vi "Verify Checksum.vi"(10 "Message ID":u8 format="%02x", 11 "Data + Checksum":string) -> (3 "Pass":bool)   [LabVIEW 2019]
doc: "Calculates what the checksum of the message should be and verifies it is correct."
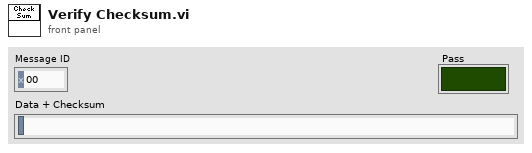
[diagram p1: front panel]
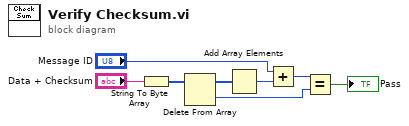
[diagram p0: block diagram]
diagram:
  n1 = String To Byte Array(string="Data + Checksum") -> (unsigned byte array=w4:u8[])
  n2 = Delete From Array(array=w4) -> (deleted portion=w7:u8, array with subset deleted=w5:u8[])  [unwired: 2 in]
  n3 = Add Array Elements(numeric array=w5) -> (sum=w6:u8)
  n4 = Add(x="Message ID", y=w6) -> (x+y=w2:u8)
  n5 = Equal?(x=w2, y=w7) -> (x = y?=→"Pass":bool)
